vi "Process (DRAM 128-Bit).vi"(0 "write data":T5, 1 "reset":bool, 2 "memory":refnum<k21>, 5 "read request":T4, 7 "arbiter configuration":T1={"write grant time (clocks)"=100, "read grant time (clocks)"=100}, 9 "Sim_DRAM Skew":fxp<+,32,0>, 12 "ready for retrieve data (T)":bool=TRUE) -> (3 "in reset":bool, 4 "retrieve data":T2, 13 "ready for read request":bool, 14 "ready for write":bool)   [LabVIEW 2012, in "FIFO.lvlib" / "niRFRIO Memory 1.0.0 FPGA.lvlib"]
uses:
  <userlib>/FPGA Library/Code Development/DRAM/RF-RIO/Memory/1.0.0/FPGA/niRFRIO Memory 1.0.0 FPGA.lvlib
  <userlib>/FPGA Library/Code Development/DRAM/RF-RIO/Memory/1.0.0/FPGA/Public/Write Data (128-Bit).ctl
  <userlib>/FPGA Library/Code Development/DRAM/RF-RIO/Memory/1.0.0/FPGA/Public/U128.ctl
  <userlib>/FPGA Library/Code Development/DRAM/RF-RIO/Memory/1.0.0/FPGA/Public/Read Request.ctl
  <userlib>/FPGA Library/Code Development/DRAM/RF-RIO/Memory/1.0.0/FPGA/Public/Retrieve Data (128-Bit).ctl
  <userlib>/FPGA Library/Code Development/DRAM/RF-RIO/Memory/1.0.0/FPGA/Public/Timeslot Arbiter Configuration.ctl
  <vilib>/rvi/DataTransferAndStorage/Container/Common/niFpgaContainerExecOnDevCompGetState.vi
  <vilib>/rvi/DataTransferAndStorage/Container/Common/niFpgaContainerGetUniqueNameForEmu.vi
  <vilib>/rvi/Memory/Memory_Emulation/niFpgaMemoryEmulationCacheClearOnFirstRun.vi
  <vilib>/rvi/Memory/Memory_Emulation/nirvimemoryEmulationManagerCache_MakeExclusive.vi
  <vilib>/rvi/Memory/Memory_Emulation/nirvimemoryEmulationManagerCache_GetValue.vi
  <vilib>/rvi/Memory/Memory_Emulation/nirvimemoryEmulationManagerCache_ReleaseExclusive.vi
  <vilib>/rvi/Memory/Memory_Emulation/nirvimemoryEmulationManagerCache_InsertValue.vi
  <vilib>/Utility/error.llb/Clear Errors.vi
  <vilib>/rvi/Memory/Memory_Emulation/nirvimemoryEmulationManagerCache_SetValue.vi
  <vilib>/rvi/Memory/Memory_Emulation/niFpgaMemoryEmulationDramWriteAndRequestDataApplyByteEnables.vi
  <vilib>/rvi/DataTransferAndStorage/Container/XNode/niFpgaContainer.xnode
  <vilib>/rvi/Memory/Memory_Emulation/niFpgaMemoryEmulationDramRetrieveDataRefIn.vi
  <vilib>/rvi/Memory/Memory_Emulation/niFpgaMemoryEmulationDramWriteAndRequestDataRefIn.vi
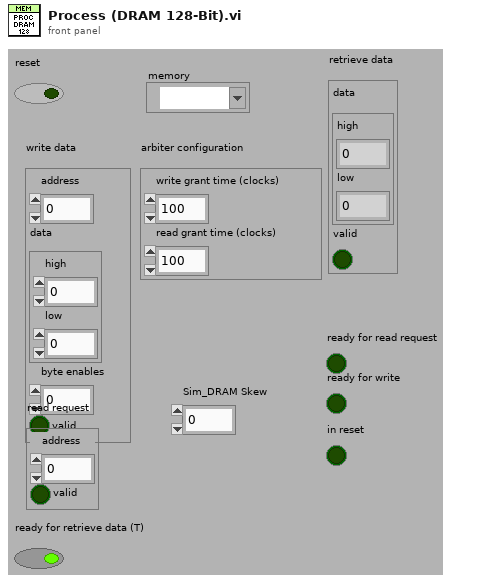
[diagram p1: front panel]
types:
  T1 = typedef "FIFO.lvlib/niRFRIO Memory 1.0.0 FPGA.lvlib/Timeslot Arbiter Configuration.ctl" = cluster{"write grant time (clocks)":u16, "read grant time (clocks)":u16}
  T2 = typedef "FIFO.lvlib/niRFRIO Memory 1.0.0 FPGA.lvlib/Retrieve Data (128-Bit).ctl" = cluster{"data":T3, "valid":bool}
  T3 = typedef "FIFO.lvlib/niRFRIO Memory 1.0.0 FPGA.lvlib/U128.ctl" = cluster{"high":u64, "low":u64}
  T4 = typedef "FIFO.lvlib/niRFRIO Memory 1.0.0 FPGA.lvlib/Read Request.ctl" = cluster{"address":u32, "valid":bool}
  T5 = typedef "FIFO.lvlib/niRFRIO Memory 1.0.0 FPGA.lvlib/Write Data (128-Bit).ctl" = cluster{"address":u32, "data":T3, "byte enables":u16, "valid":bool}
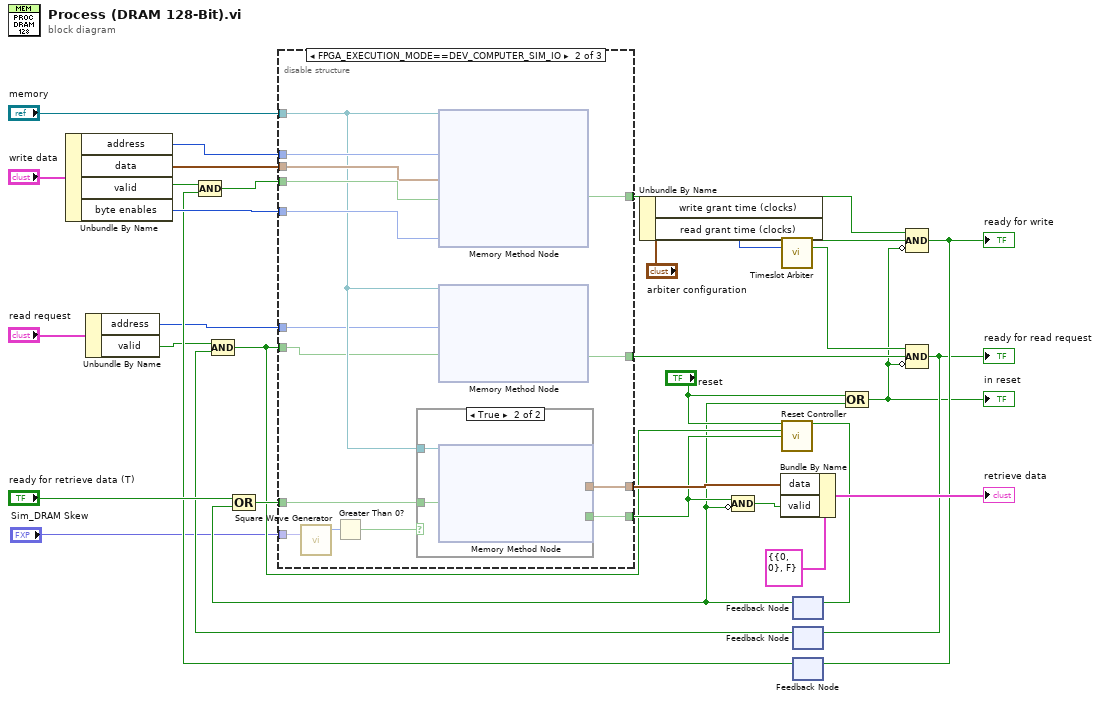
[diagram p0: block diagram]
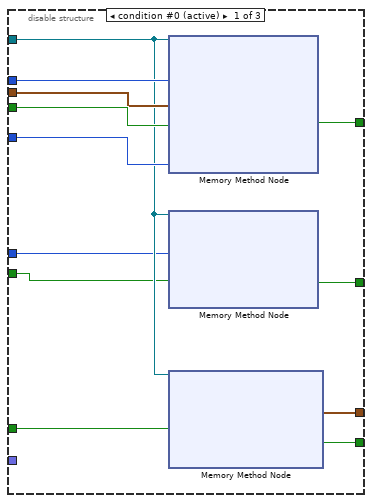
[diagram p2: hidden frame]
diagram:
  n1 = Unbundle By Name("write data") -> ("address"=w27:u32, "data"=w26:T3, "valid"=w25:bool, "byte enables"=w28:u16)
  n2 = Unbundle By Name("read request") -> ("address"=w15:u32, "valid"=w14:bool)
  n3 = Unbundle By Name("arbiter configuration") -> ("write grant time (clocks)"=w3:u16, "read grant time (clocks)"=w2:u16)
  n4 = call <userlib>:"Timeslot Arbiter.vi"("write grant time (clocks)"=w3, "read grant time (clocks)"=w2) -> ("write"=w31:bool, "read"=w12:bool)  [unwired: 12 in]
  n5 = feedback #1() -> (w6:bool)  [unwired: 1 in]
  n6 = Compound Arithmetic op=OR("ready for retrieve data (T)", w6) -> (w33:bool)
  n7 = feedback #2() -> (w9:bool)  [unwired: 1 in]
  n8 = Compound Arithmetic op=AND(w14, w9) -> (w13:bool)
  n9 = feedback #3() -> (w17:bool)  [unwired: 1 in]
  n10 = Compound Arithmetic op=AND(w25, w17) -> (w29:bool)
  n11 = disable-structure shown="FPGA_EXECUTION_MODE==DEV_COMPUTER_SIM_IO" {
    disable-tunnel: w33 -> [w46 w61 _]
    disable-tunnel: [w45 w60 _] -> w32
    disable-tunnel: w29 -> [w44 w59 _]
    disable-tunnel: w28 -> [w43 w58 _]
    disable-tunnel: w27 -> [w42 w57 _]
    disable-tunnel: w26 -> [w41 w56 _]
    disable-tunnel: "memory" -> [w40 w55 _]
    disable-tunnel: [w39 w54 _] -> w21
    disable-tunnel: [w38 w53 _] -> w20
    disable-tunnel: w15 -> [w37 w52 _]
    disable-tunnel: w13 -> [w36 w51 _]
    disable-tunnel: [w35 w50 _] -> w11
    disable-tunnel: "Sim_DRAM Skew" -> [_ w48 _]
    frame condition #0 (active) {
      n12 = xnode ("Memory Method Node")("Address"=w42, "Data"=w41, "Input Valid"=w44, "Byte Enables"=w43, "Memory In"=w40) -> ("Ready for Input"=w45:bool)  [unwired: 1 out]
      n13 = xnode ("Memory Method Node")("Address"=w37, "Input Valid"=w36, "Memory In"=w40) -> ("Ready for Input"=w35:bool)  [unwired: 1 out]
      n14 = xnode ("Memory Method Node")("Ready for Output"=w46, "Memory In"=w40) -> ("Data"=w39:cluster{"high":u64, "low":u64}, "Output Valid"=w38:bool)  [unwired: 1 out]
    }
    frame condition #1 {
      n15 = call "Square Wave Generator"("phase offset (periods)"=w48) -> ("square wave out"=w49:i16)  [unwired: 14 in]
      n16 = Greater Than 0?(x=w49) -> (x > 0?=w47:bool)
      n17 = case shown="True" w47 {
        tunnel: w61 -> [_ w65]
        tunnel: w55 -> [_ w64]
        tunnel: [_ w63] -> w54
        tunnel: [_ w62] -> w53
        frame False {
        }
        frame True {
          n18 = xnode ("Memory Method Node")("Ready for Output"=w65, "Memory In"=w64) -> ("Data"=w63:cluster{"high":u64, "low":u64}, "Output Valid"=w62:bool)  [unwired: 1 out]
        }
      }
      n19 = xnode ("Memory Method Node")("Address"=w57, "Data"=w56, "Input Valid"=w59, "Byte Enables"=w58, "Memory In"=w55) -> ("Ready for Input"=w60:bool)  [unwired: 1 out]
      n20 = xnode ("Memory Method Node")("Address"=w52, "Input Valid"=w51, "Memory In"=w55) -> ("Ready for Input"=w50:bool)  [unwired: 1 out]
    }
    frame condition #2 {
    }
  }
  n21 = Compound Arithmetic op=AND(w20, invert w6) -> (w22:bool)
  n22 = Bundle By Name(cluster=T2 {"data"={"high"=0, "low"=0}, "valid"=FALSE} ("retrieve data"), "data"=w21, "valid"=w22) -> (→"retrieve data":T2)
  n23 = call <userlib>:"Reset Controller.vi"("reset"="reset", "issued read request"=w13, "retrieved data"=w20) -> ("flushing memory pipe"=w7:bool)  [unwired: 12 in]
  n24 = feedback-in #1(w7) -> ()
  n25 = Compound Arithmetic op=OR("reset", w6) -> (w5:bool)
  "in reset" <- w5
  n26 = Compound Arithmetic op=AND(w32, w31, invert w5) -> (w18:bool)
  "ready for write" <- w18
  n27 = feedback-in #3(w18) -> ()
  n28 = Compound Arithmetic op=AND(w12, w11, invert w5) -> (w10:bool)
  "ready for read request" <- w10
  n29 = feedback-in #2(w10) -> ()
